vi "Load or create a cfg.vi"(8 "error in":errorcluster, 10 "Tree Refnum":refnum<vi>, 11 "Tbl Refnum in":refnum<vi>) -> (0 "error out":errorcluster, 1 "cfg file refnum out":refnum<file>, 2 "Tree Refnum out":refnum<vi>, 3 "Tbl Refnum out":refnum<vi>)   [LabVIEW 2010]
uses:
  <vilib>/Utility/miscctls.llb/LVRowAndColumnTypeDef.ctl
panel:
  out "All Tags":string[](array[string])
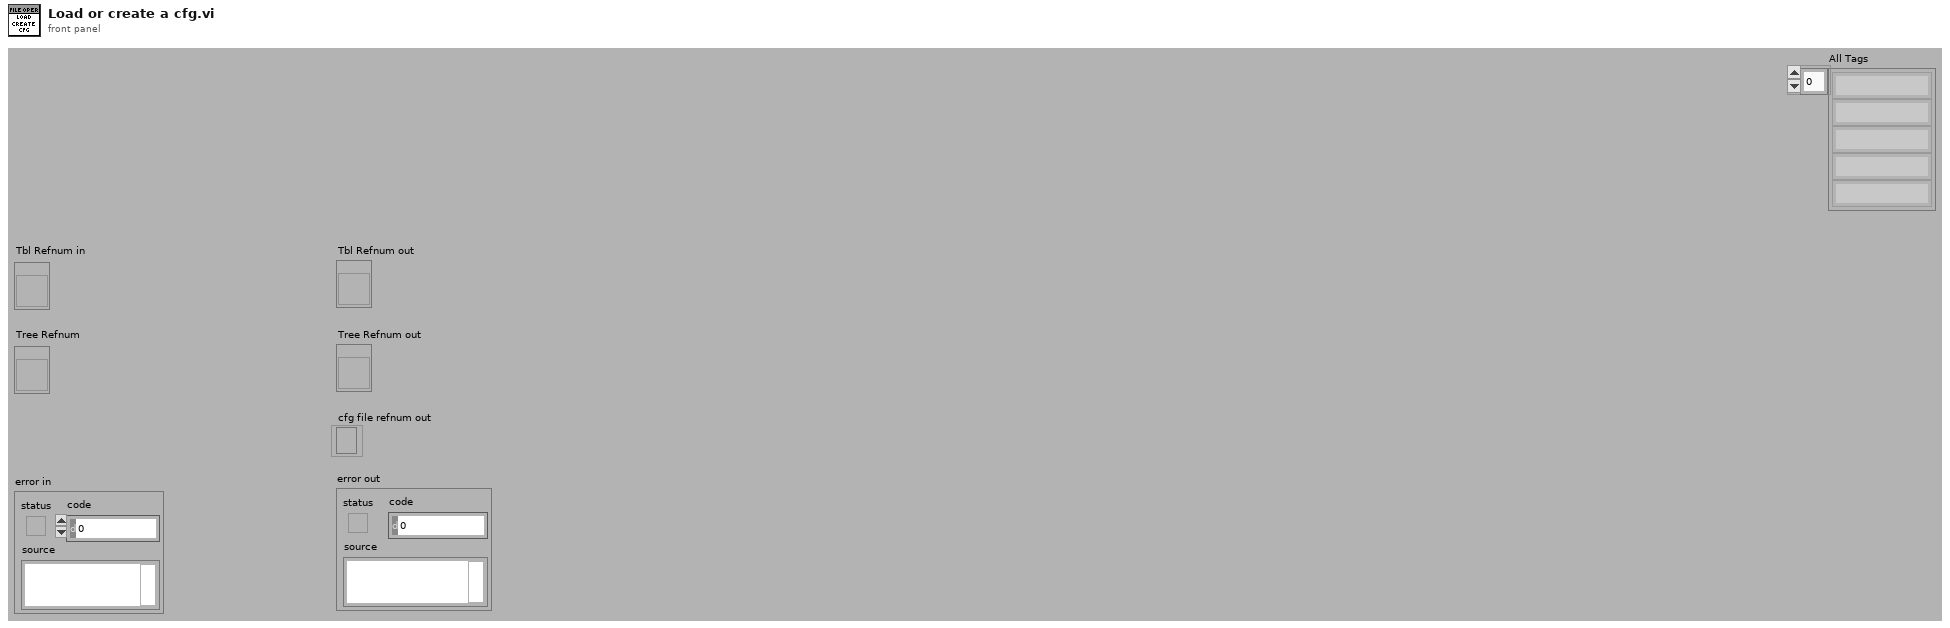
[diagram p1: front panel]
types:
  T1 = typedef "LVRowAndColumnTypeDef.ctl" = cluster{"Row":i32, "Column":i32}
  T2 = enum16{"open", "replace", "create", "open or create", "replace or create", "replace or create with confirmation"}
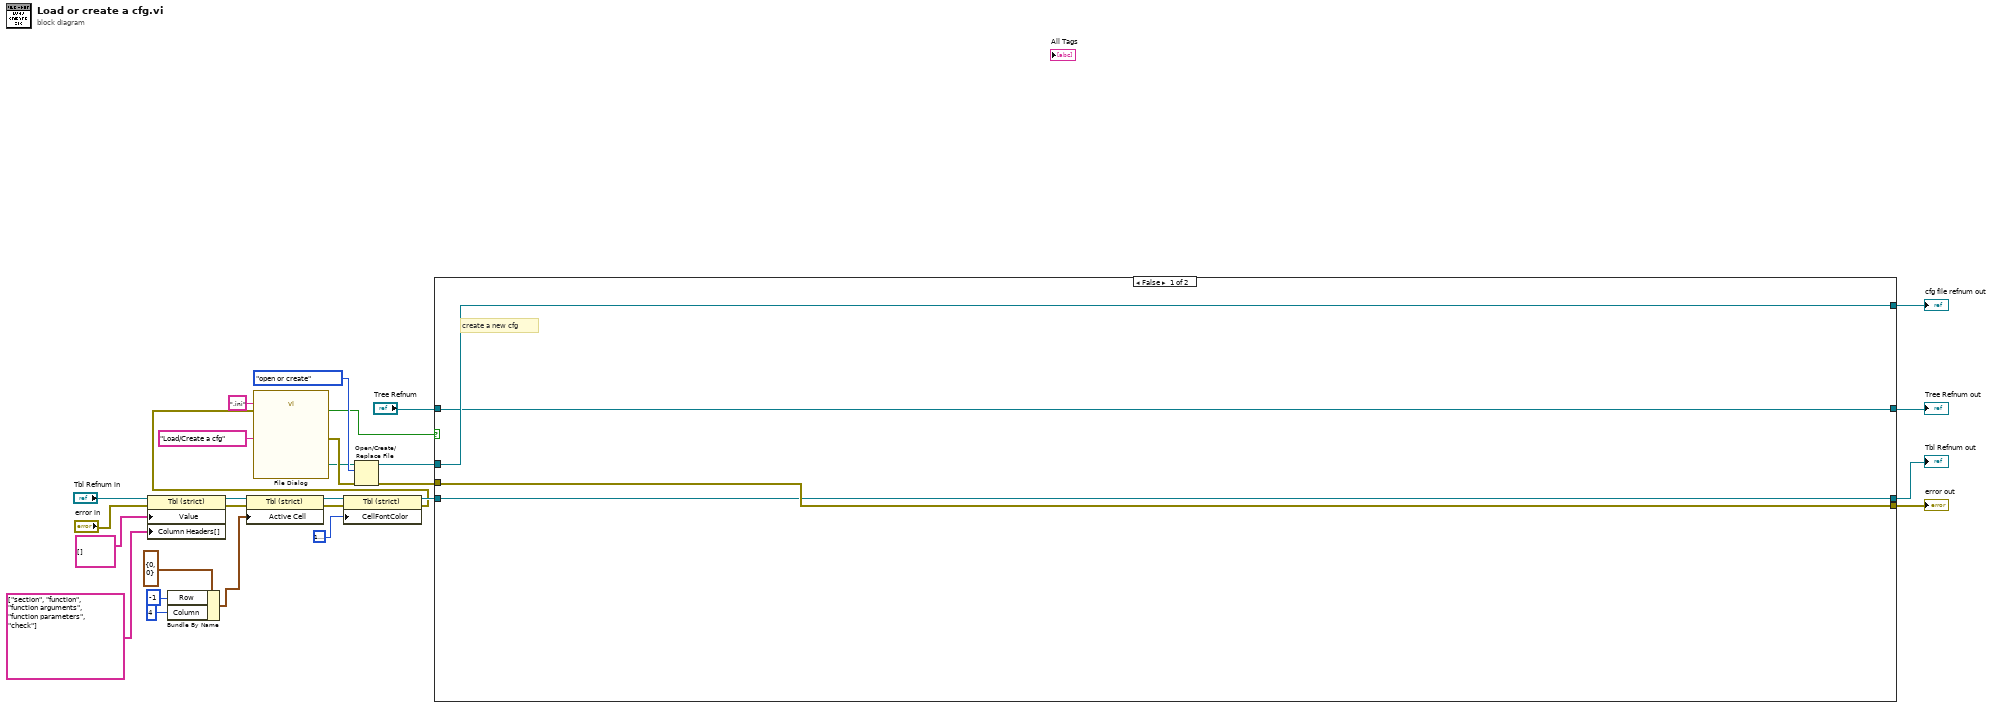
[diagram p0: block diagram]
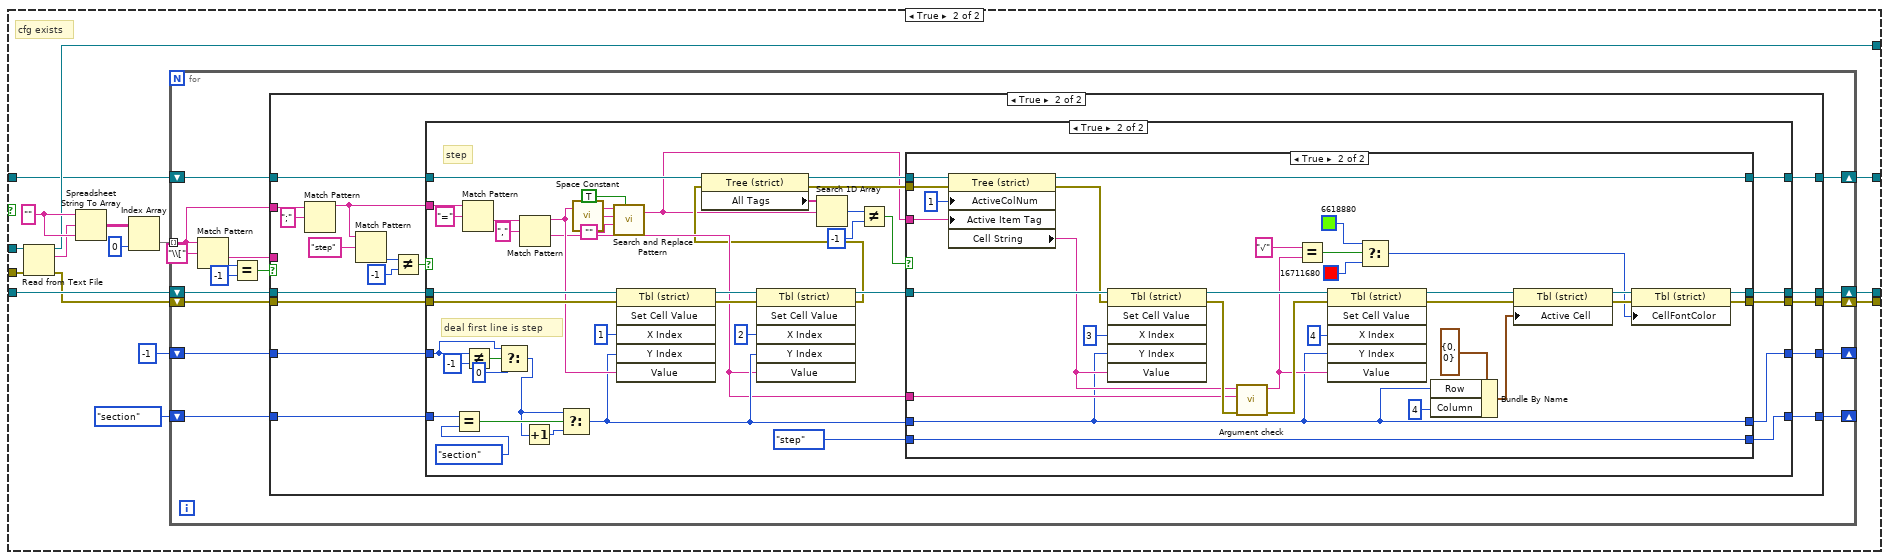
[diagram p2: hidden frame]
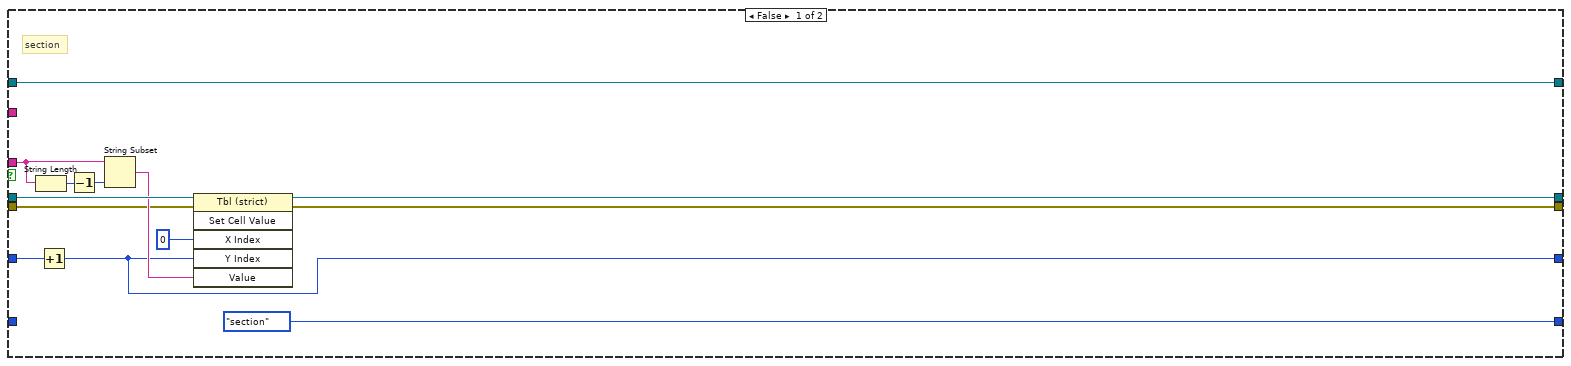
[diagram p3: hidden frame]
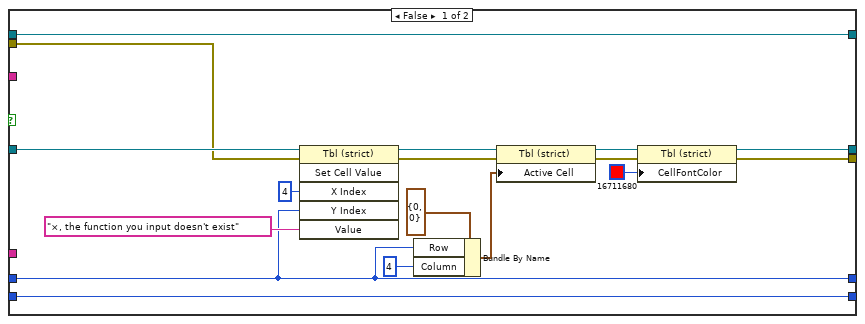
[diagram p5: hidden frame]
diagram:
  n1 = property class="Tbl (strict)"(reference="Tbl Refnum in", error in="error in", "Value"=string[][] [], "Column Headers[]"=string[] ["section", "function", "function arguments", "function parameters", "check"] ("Row Header Strings[]")) -> (reference out=w11:refnum<vi>, error out=w10:errorcluster)
  n2 = Bundle By Name(cluster=T1 {"Row"=0, "Column"=0} ("Active Cell:Active Cell"), "Row"=-1, "Column"=4) -> (w6:T1)
  n3 = property on="Property Node" class="Tbl (strict)"(reference=w11, error in=w10, "Active Cell"=w6) -> (reference out=w5:refnum<vi>, error out=w4:errorcluster)
  n4 = property on="Property Node" class="Tbl (strict)"(reference=w5, error in=w4, "CellFontColor"=u32 16777222) -> (reference out=w3:refnum<vi>, error out=w2:errorcluster)
  n5 = call "File Dialog"("prompt"="Load/Create a cfg", "default name"=".ini", "error in"=w2) -> ("selected path"=w26:path, "exists"=w25:bool, "error out"=w27:errorcluster)  [unwired: 9 in, 1 out]
  n6 = Open/Create/Replace File(file path (use dialog)=w26, error in=w27, operation (0:open)=T2."open or create") -> (refnum out=w24:refnum<file>, error out=w23:errorcluster)  [unwired: 3 in, 1 out]
  n7 = case shown="False" w25 {
    tunnel: w24 -> [w32 w44]
    tunnel: w23 -> [w31 w43]
    tunnel: w3 -> [w30 w41]
    tunnel: [w32 w38] -> w17
    tunnel: [w31 w37] -> w16
    tunnel: [w30 w35] -> w15
    tunnel: "Tree Refnum" -> [w29 w34]
    tunnel: [w29 w33] -> w13
    frame False {
      # "create a new cfg"
    }
    frame True {
      w46 = ""
      # "cfg exists"
      n8 = Read from Text File(file (use dialog)=w44, error in=w43) -> (refnum out=w38:refnum<file>, text=w45:string, error out=w36:errorcluster)  [unwired: 2 in, 1 out]
      n9 = Spreadsheet String To Array(format string=w46, spreadsheet string=w45, array type (2D Dbl)=w46) -> (array=w47:string[][])  [unwired: 1 in]
      n10 = Index Array(array=w47, index (col)=0 ("disabled index (col)")) -> (element=w42:string[])  [unwired: 1 in]
      n11 = for {
        tunnel: w42 -> [w58] mode=indexing
        shift-right: [w56] -> _
        shift-left: -1 -> [w60]
        shift-right: [w55] -> _
        shift-left: enum16{"section", "step"}."section" -> [w54]
        shift-right: [w53] -> w37
        shift-left: w36 -> [w52]
        shift-right: [w51] -> w35
        shift-left: w41 -> [w57]
        shift-right: [w49] -> w33
        shift-left: w34 -> [w50]
        n12 = Match Pattern(string=w58, regular expression="\\[") -> (after substring=w59:string, offset past match=w63:i32)  [unwired: 1 in, 2 out]
        n13 = Equal?(x=w63, y=-1) -> (x = y?=w61:bool)
        n14 = case shown="True" w61 {
          tunnel: w60 -> [w71 w89]
          tunnel: [w70 w88] -> w56
          tunnel: w59 -> [w77 _]
          tunnel: w58 -> [_ w82]
          tunnel: w57 -> [w74 w90]
          tunnel: [enum16{"section", "step"}."section" w87] -> w55
          tunnel: w54 -> [_ w86]
          tunnel: w52 -> [w68 w85]
          tunnel: [w67 w84] -> w53
          tunnel: [w66 w83] -> w51
          tunnel: w50 -> [w65 w79]
          tunnel: [w65 w78] -> w49
          frame False {
            # "section"
            n15 = String Length(string=w77) -> (length=w76:i32)
            n16 = Increment(x=w71) -> (x+1=w70:i32)
            n17 = Decrement(x=w76) -> (x-1=w75:i32)
            n18 = String Subset(string=w77, length (rest)=w75) -> (substring=w72:string)  [unwired: 1 in]
            n19 = invoke class="Tbl (strict)" method="Set Cell Value"(reference=w74, error in=w68, "X Index"=u32 0 ("Y Index"), "Y Index"=w70, "Value"=w72) -> (reference out=w66:refnum<vi>, error out=w67:errorcluster)  [unwired: 1 in, 4 out]
          }
          frame True {
            n20 = Match Pattern(string=w82, regular expression=";") -> (before substring=w80:string)  [unwired: 1 in, 3 out]
            n21 = Match Pattern(string=w80, regular expression="step") -> (offset past match=w92:i32)  [unwired: 1 in, 3 out]
            n22 = Not Equal?(x=w92, y=-1) -> (x != y?=w94:bool)
            n23 = case shown="True" w94 {
              tunnel: w80 -> [_ w139]
              tunnel: w90 -> [w96 w131]
              tunnel: w89 -> [w99 w102]
              tunnel: [w99 w114] -> w88
              tunnel: [w98 w115] -> w87
              tunnel: w86 -> [w98 w137]
              tunnel: w85 -> [w97 w130]
              tunnel: [w97 w119] -> w84
              tunnel: [w96 w120] -> w83
              tunnel: w79 -> [w95 w112]
              tunnel: [w95 w125] -> w78
              frame False {
                # "blank"
              }
              frame True {
                # "deal first line is step"
                # "step"
                n24 = Equal?(x=w137, y=enum16{"section", "step"}."section") -> (x = y?=w136:bool)
                n25 = Match Pattern(string=w139, regular expression="=") -> (after substring=w133:string)  [unwired: 1 in, 3 out]
                n26 = Not Equal?(x=w102, y=-1) -> (x != y?=w103:bool)
                n27 = Select(t=w102, s=w103, f=0) -> (s? t:f=w100:i32)
                n28 = Match Pattern(string=w133, regular expression=",") -> (before substring=w124:string, after substring=w117:string)  [unwired: 1 in, 2 out]
                n29 = Increment(x=w100) -> (x+1=w135:i32)
                n30 = Select(t=w100, s=w136, f=w135) -> (s? t:f=w118:i32)
                n31 = call <vilib>:"Space Constant.vi"() -> ("String"=w123:string)
                n32 = call <vilib>:"Search and Replace Pattern.vi"("string"=w124, "regular expression (\"\")"=w123, "replace string (\"\")"="", "replace all? (F)"=TRUE) -> ("result string"=w105:string)  [unwired: 1 in, 1 out]
                n33 = invoke class="Tbl (strict)" method="Set Cell Value"(reference=w131, error in=w130, "X Index"=u32 1, "Y Index"=w118, "Value"=w124) -> (reference out=w128:refnum<vi>, error out=w129:errorcluster)  [unwired: 1 in, 4 out]
                n34 = invoke class="Tbl (strict)" method="Set Cell Value"(reference=w128, error in=w129, "X Index"=u32 2, "Y Index"=w118, "Value"=w117) -> (reference out=w126:refnum<vi>, error out=w110:errorcluster)  [unwired: 1 in, 4 out]
                n35 = property on="Property Node" class="Tree (strict)"(reference=w112, error in=w110) -> (reference out=w111:refnum<vi>, error out=w106:errorcluster, "All Tags"=w113:string[])
                n36 = Search 1D Array(1D array=w113, element=w105) -> (index of element=w109:i32)  [unwired: 1 in]
                n37 = Not Equal?(x=w109, y=-1) -> (x != y?=w107:bool)
                n38 = case shown="True" w107 {
                  tunnel: w126 -> [w155 w188]
                  tunnel: [w149 w184] -> w125
                  tunnel: w111 -> [w149 w183]
                  tunnel: w106 -> [w154 w182]
                  tunnel: w105 -> [_ w181]
                  tunnel: [w142 w159] -> w120
                  tunnel: [w141 w160] -> w119
                  tunnel: w118 -> [w144 w164]
                  tunnel: w117 -> [_ w176]
                  tunnel: enum16{"section", "step"}."step" -> [w148 w174]
                  tunnel: [w148 w174] -> w115
                  tunnel: [w144 w164] -> w114
                  frame False {
                    n39 = invoke class="Tbl (strict)" method="Set Cell Value"(reference=w155, error in=w154, "X Index"=u32 4, "Y Index"=w144, "Value"="×, the function you input doesn't exist") -> (reference out=w153:refnum<vi>, error out=w152:errorcluster)  [unwired: 1 in, 4 out]
                    n40 = Bundle By Name(cluster=T1 {"Row"=0, "Column"=0} ("Active Cell:Active Cell"), "Row"=w144, "Column"=4) -> (w147:T1)
                    n41 = property on="Property Node" class="Tbl (strict)"(reference=w153, error in=w152, "Active Cell"=w147) -> (reference out=w146:refnum<vi>, error out=w145:errorcluster)
                    n42 = property on="Property Node" class="Tbl (strict)"(reference=w146, error in=w145, "CellFontColor"=u32 16711680) -> (reference out=w142:refnum<vi>, error out=w141:errorcluster)
                  }
                  frame True {
                    n43 = property class="Tree (strict)"(reference=w183, error in=w182, "ActiveColNum"=1 ("Active Cell:Active Column Number"), "Active Item Tag"=w181) -> (reference out=w184:refnum<vi>, error out=w185:errorcluster, "Cell String"=w175:string)
                    n44 = invoke class="Tbl (strict)" method="Set Cell Value"(reference=w188, error in=w185, "X Index"=u32 3, "Y Index"=w164, "Value"=w175) -> (reference out=w180:refnum<vi>, error out=w178:errorcluster)  [unwired: 1 in, 4 out]
                    n45 = call "Argument check.vi"("error in"=w178, "Arg"=w176, "par"=w175) -> ("error out"=w177:errorcluster, "Check result"=w169:string)  [unwired: 6 in, 1 out]
                    n46 = Equal?(x="√", y=w169) -> (x = y?=w167:bool)
                    n47 = invoke class="Tbl (strict)" method="Set Cell Value"(reference=w180, error in=w177, "X Index"=u32 4, "Y Index"=w164, "Value"=w169) -> (reference out=w173:refnum<vi>, error out=w172:errorcluster)  [unwired: 1 in, 4 out]
                    n48 = Select(t=u32 6618880, s=w167, f=u32 16711680) -> (s? t:f=w158:u32)
                    n49 = Bundle By Name(cluster=T1 {"Row"=0, "Column"=0} ("Active Cell:Active Cell"), "Row"=w164, "Column"=4) -> (w163:T1)
                    n50 = property on="Property Node" class="Tbl (strict)"(reference=w173, error in=w172, "Active Cell"=w163) -> (reference out=w162:refnum<vi>, error out=w161:errorcluster)
                    n51 = property on="Property Node" class="Tbl (strict)"(reference=w162, error in=w161, "CellFontColor"=w158) -> (reference out=w159:refnum<vi>, error out=w160:errorcluster)
                  }
                }
              }
            }
          }
        }
      }
    }
  }
  "error out" <- w16
  "cfg file refnum out" <- w17
  "Tbl Refnum out" <- w15
  "Tree Refnum out" <- w13
